vi "AK Befehl Auswerten_v1.3.vi"(10 "Array":string[](array[string])) -> (2 "String für schreiben":string)   [LabVIEW 2020, in "AK-Schnittstelle.lvlib"]
uses:
  AK-Schnittstelle.lvlib
  Aktionen Stoernummern pruefen.ctl
  Aktionen Zustandsfehlerinformation.ctl
  AK Namen Aktionen.ctl
  Seiten/FT-IR/Aktion FGV Rezepte wechseln.ctl
  Seiten/FT-IR/AK-manuell.ctl
  Seiten/System Einstellungen V2/Aktioen FGV System Konstanten.ctl
  Aktionen Gespeicherte Werte.ctl
  Seiten/System Einstellungen V2/Aktioen FGV System.ctl
  Funktionstasten/Funktionstasten-Aktion.ctl
  Funktionstasten/Zustaende.ctl
  Schedule Modul/Aktion FGV Scheduler Status.ctl
  Seiten/FT-IR/FGV FT-IR Aktionen.ctl
  Seiten/FT-IR/FGV FT-IR Diagnose Aktionen.ctl
  Seiten/Erweiterte Konfig/Status Dichtheitstest Aktionen.ctl
  Seiten/Erweiterte Konfig/FGV PID Aktionen.ctl
  Seiten/Anlagengrenzwerte/FGV Anlagengrenzwerte Aktionen.ctl
  Funktionstasten/Betriebsart.ctl
  Seiten/Log Konfig/Aktionen Trigger.ctl
  Messdaten/Aktionen FGV Messdaten.ctl
  Seiten/FT-IR/TOOLweb Interface Library/TOOLweb Rezept wechseln.vi
  Seiten/Erweiterte Konfig/Dichtheitstest.vi
  Funktionstasten/Funktionstasten.lvlib
  Seiten/Log Konfig/LogKonfig.lvlib
  Seiten/FT-IR/FT-IR.lvlib
  Seiten/FT-IR/FGV FT-IR Gasliste Aktionen.ctl
  Messdaten/Messdaten.lvlib
  Seiten/System Einstellungen V2/System Einstellungen V2.lvlib
  Seiten/Erweiterte Konfig/Erweiterte Konfig.lvlib
  Allgemein/allgemeine Sub-VIs.lvlib
  cRIO/PC/Kommunikation mit cRIO.lvlib
  Seiten/Anlagengrenzwerte/Anlagengrenzwerte.lvlib
  Seiten/FT-IR/TOOLweb Interface Library/TOOLweb Interface.lvlib
  Schedule Modul/Schedule Modul.lvlib
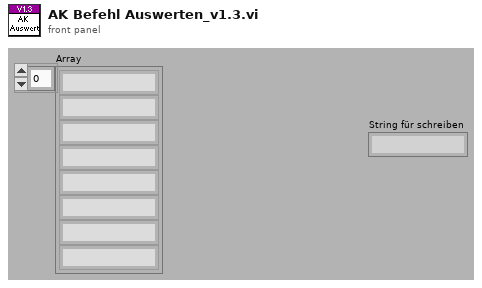
[diagram p1: front panel]
types:
  T1 = typedef "AK-Schnittstelle.lvlib/Aktionen Stoernummern pruefen.ctl" = enum16{"lesen", "prüfen"}
  T2 = typedef "AK-Schnittstelle.lvlib/Aktionen Zustandsfehlerinformation.ctl" = enum16{"OK", "Offline", "Busy", "Syntax Error", "Datenfehler"}
  T3 = typedef "AK-Schnittstelle.lvlib/AK Namen Aktionen.ctl" = enum16{"lesen", "laden", "speichern Namen", "AK Namen", "Liste erstellen", "EKFG erstellen", "speichern EKFG", "EKFG schreiben", "Neuen Eintrag erzeugen"}
  T4 = typedef "FT-IR.lvlib/AK-manuell.ctl" = enum16{"manuell", "Diesel", "CNG", "Gasoline"}
  T5 = typedef "FT-IR.lvlib/Aktion FGV Rezepte wechseln.ctl" = enum16{"lesen", "Rezepte", "Rezeptindex", "Diesel", "Gasoline", "NCG", "laden", "speichern", "AK/Man"}
  T6 = typedef "System Einstellungen V2.lvlib/Aktioen FGV System Konstanten.ctl" = enum16{"lesen", "laden", "speichern", "Sprache"}
  T7 = typedef "System Einstellungen V2.lvlib/Aktioen FGV System.ctl" = enum16{"lesen", "laden", "speichern", "Optionen schreiben", "Zeitstempel", "Reset BMP", "Reset SQP", "Wartung", "Werkseinstellung"}
  T8 = typedef "AK-Schnittstelle.lvlib/Aktionen Gespeicherte Werte.ctl" = enum16{"lesen", "laden", "speichern", "Seriell", "TCP", "Diverse", "AKTIV", "AK-Namen"}
  T9 = typedef "Messdaten.lvlib/Aktionen FGV Messdaten.ctl" = enum16{"lesen", "schreiben", "löschen", "Mittelwerte", "Komponente"}
  T10 = typedef "Funktionstasten.lvlib/Zustaende.ctl" = enum16{"Standby", "Pause", "Eco", "Messen", "Kalibrieren", "Spülen Filter", "Spülen Leitung", "Umgebungsluft", "0-Gas", "Cal-Gas", "CG zu PNS", "-------------", "Init 1", "Init 2", "Init 3", "Init 4", "Messen vorbereiten", "Messen durchführen", "Exit"}
  T11 = typedef "Funktionstasten.lvlib/Funktionstasten-Aktion.ctl" = enum16{"Initialisieren", "Zustand setzen", "Taste gedrückt", "Fehler speichern", "Lesen", "Manuell", "Remote", "Bitparallel", "Samplepoint", "Zeit Prüfen", "reset Umschalten"}
  T12 = typedef "Schedule Modul.lvlib/Aktion FGV Scheduler Status.ctl" = enum16{"lesen", "init", "aktiv", "inaktiv"}
  T13 = typedef "FT-IR.lvlib/FGV FT-IR Aktionen.ctl" = enum16{"lesen", "NOG setzen", "NOS setzen", "Initialisieren", "speichern", "ALLES setzen", "FT-IR Spektrum loggen", "Komm Stoppen", "Spektrum LogKonfig"}
  T14 = typedef "FT-IR.lvlib/FGV FT-IR Gasliste Aktionen.ctl" = enum16{"lesen", "Gasliste FT-IR", "Gasliste ausgelesen", "laden", "speichern", "löschen"}
  T15 = typedef "FT-IR.lvlib/FGV FT-IR Diagnose Aktionen.ctl" = enum16{"Lesen", "Diagnose Schreiben", "Min Schreiben", "Max Schreiben"}
  T16 = typedef "Erweiterte Konfig.lvlib/Status Dichtheitstest Aktionen.ctl" = enum16{"lesen", "Zeitstempel", "Daten", "läuft", "Protokolldaten"}
  T17 = typedef "Erweiterte Konfig.lvlib/FGV PID Aktionen.ctl" = enum16{"Lesen", "Schreiben PID", "Schreiben Sonstige", "Dichtheitstest", "Aktionen Dicht.", "Parameter Sensor"}
  T18 = typedef "Anlagengrenzwerte.lvlib/FGV Anlagengrenzwerte Aktionen.ctl" = enum16{"Lesen", "Grenzwerte schreiben"}
  T19 = typedef "Funktionstasten.lvlib/Betriebsart.ctl" = enum16{"Manuell", "Remote", "Bitparallel"}
  T20 = typedef "LogKonfig.lvlib/Aktionen Trigger.ctl" = enum16{"lesen", "ALLE schreiben", "Trigger prüfen", "Trigger rücksetzen"}
  T21 = cluster{"Modell":string, "ProjektNummer":string, "Software Version":string, "Seriennummer":string}
  T22 = typedef "System Einstellungen V2.lvlib/Optionen.ctl" = cluster{"Störmeldep.":bool, "Betriebszustände":bool, "AK in ppm":bool, "log Cal-Gas":bool, "log 0-Gas":bool, "Durchflusssensor 0-5V":bool, "PNS?":bool, "Mit N2 spülen":bool, "TRE08":bool, "Amium 10-Fach":bool, "Verticale Scrollbar aktiv":bool, "Loggingtakt":bool, "AK Rezeptwechsel gleich wie MKS":bool, "NG ECO":bool}
  T23 = typedef "AK-Schnittstelle.lvlib/Diverse gespeicherte Werte.ctl" = cluster{"Kalibriergaseingang":i16, "SamplePoint":i16, "CalGas zu PNS":i16, "Gas-Reihenfolge":i16[], "Zeit 0-Gas":sgl, "Zeit CalGas":sgl, "AK Befehlssatz":T24}
  T24 = typedef "AK-Schnittstelle.lvlib/AK Befehlssatz.ctl" = enum16{"MEXA", "IAG v1.4", "AVL (Puma)", "PEUS"}
  T25 = typedef "String - Ausgabefeld.ctl" = string
  T26 = typedef "Verwaltung - cRIO.lvlib/TC Eingaenge.ctl" = cluster{"TC0: Reserve":sgl, "TC1: HL zu FT-IR":sgl, "TC2: HL Extern SP1":sgl, "TC3: HL Extern SP2":sgl, "TC4: Reserve":sgl, "TC5: Reserve":sgl, "TC6: Reserve":sgl, "TC7: Reserve":sgl, "TC8: FT-IR":sgl, "TC9: Reserve":sgl, "TC10: Schaltschrank":sgl, "TC11: Umgebung":sgl}
  T27 = typedef "Verwaltung - cRIO.lvlib/Analog Eingaenge.ctl" = cluster{"AI0: Durchfluss FT-IR":sgl, "AI1: Druck Ausgang":sgl, "AI2: Umgebungsdruck":sgl, "AI3: Druck FT-IR":sgl, "AI4: Druck CalGas":sgl, "AI5: Reserve":sgl, "AI6: Reserve":sgl, "AI7: Reserve":sgl, "Rohwert Durchfluss FT-IR":sgl, "Rohwert Druck Ausgang":sgl, "Rohwert Umgebungsdruck":sgl, "Rohwert Druck FT-IR":sgl, "Rohwert Druck CalGas":sgl, "Rohwert AI5":sgl, "Rohwert AI6":sgl, "Rohwert AI7":sgl, "Rohwert Diffdruck mbar FTIR":sgl}
  T28 = typedef "Erweiterte Konfig.lvlib/Sonstige Parameter.ctl" = cluster{"Lüfter langsam":sgl, "Lüfter schnell":sgl, "FT-IR Kühlung Soll":sgl, "FT-IR Kühlung Max":sgl, "Überwachung":T29, "Befüllung aktiv":T30, "Stickstoff Befüllzeit":sgl, "Befüllintervall":sgl, "Kalibrierwert FT-IR":sgl, "Offset Ausgang":sgl, "Offset FT-IR":sgl, "Offset Druck FT-IR":sgl, "Dichtheitstest Zeit":sgl, "Dichtheitstest Abfall":sgl, "Dichtheitstest Umfang":T31, "Offset Umgebung":sgl, "Max Taupunkt":sgl, "Pumpendrehzahl":sgl, "ext. Befüllung":T30, "Ext. Stickstoff Befüllzeit":sgl}
  T29 = typedef "Auswahlfeld.ctl" = u16
  T30 = typedef "LogKonfig.lvlib/Auswahlfeld aktiviert-deaktiviert.ctl" = u16
  T31 = typedef "Erweiterte Konfig.lvlib/Dichtheitstest Umfang.ctl" = u16
  T32 = typedef "Anlagengrenzwerte.lvlib/Anlagen-Grenzwerte Anzeige.ctl" = cluster{"Eingangsdruck FT-IR:":T33, "Durchfluss FT-IR:":T33, "Durchfluss CalGas:":T33, "Druck Ausgang:":T33, "Druck Kalter Block:":T33, "Heizleitungen intern:":T33, "Heizleitung zu FT-IR:":T33, "Heizung Filterblock:":T33, "Heizung Pumpe:":T33, "Heizleitung Extern SP1:":T33, "Heizleitung Extern SP2:":T33, "FT-IR Heizung Messzelle:":T33, "Schaltschranktemperatur:":T33, "Gaskühler:":T33}
  T33 = typedef "Anlagengrenzwerte.lvlib/Anlagen-Parameter Anzeige.ctl" = cluster{"Sollwert":sgl, "Warn-Min":sgl, "Warn-Max":sgl, "Abschalt-Min":sgl, "Abschalt-Max":sgl, "Regler":u16}
  T34 = typedef "LogKonfig.lvlib/Element Triggerereignisse.ctl" = cluster{"Trigger verwenden":T30, "Messwert":u16, "kl./gr.":u16, "Wert":sgl, "Puffergröße":sgl}
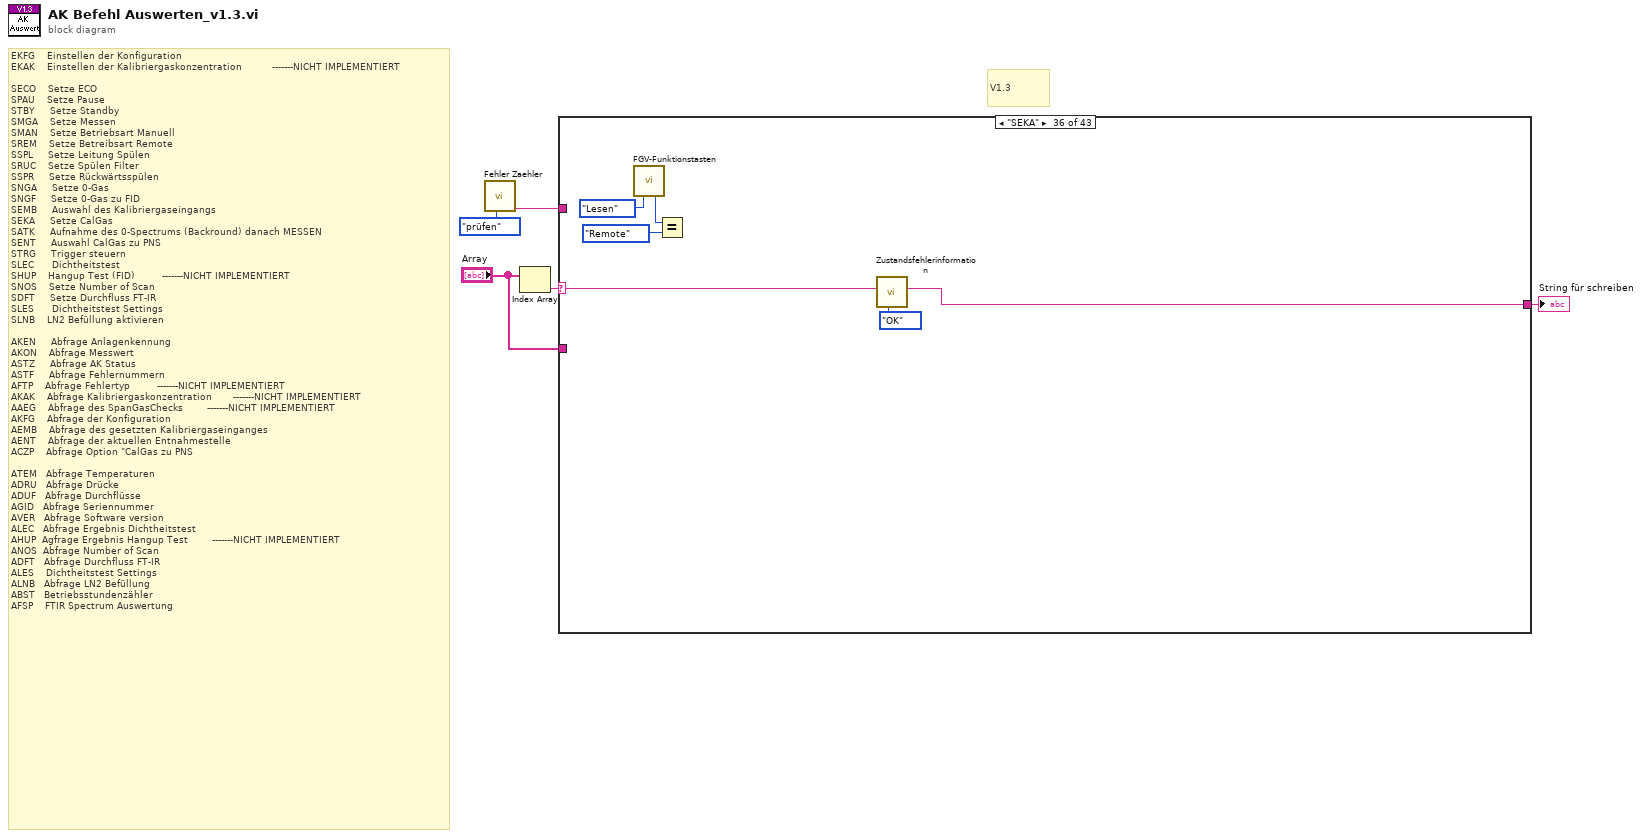
[diagram p0: block diagram]
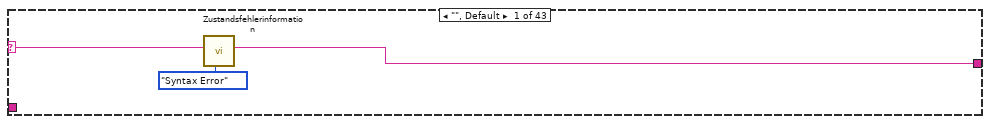
[diagram p2: hidden frame]
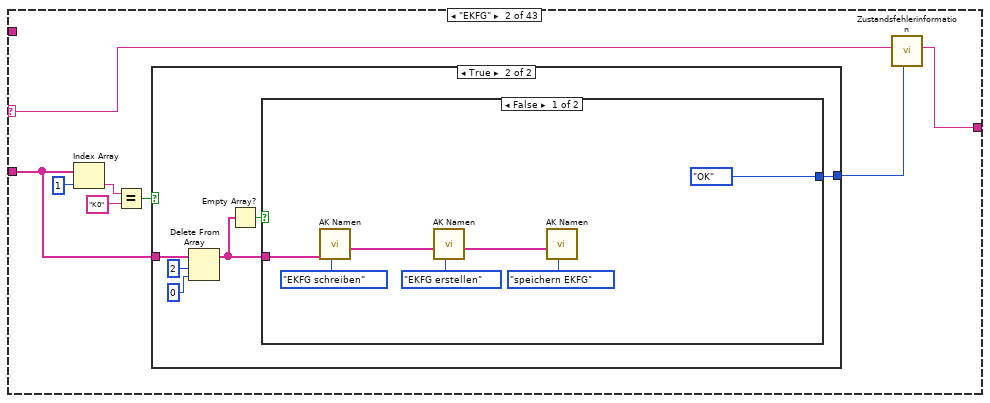
[diagram p3: hidden frame]
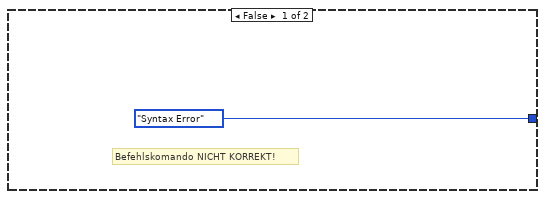
[diagram p4: hidden frame]
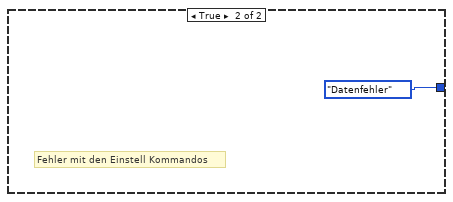
[diagram p5: hidden frame]
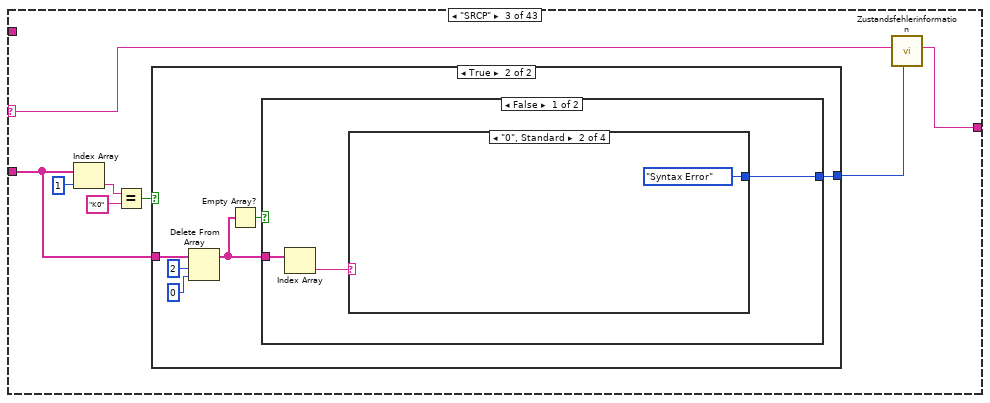
[diagram p6: hidden frame]
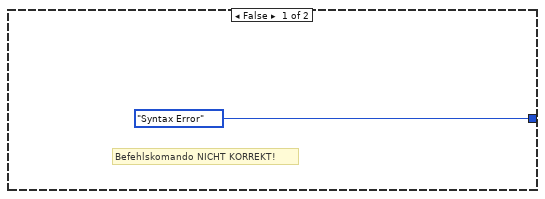
[diagram p7: hidden frame]
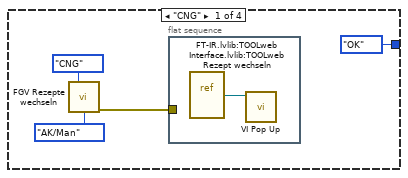
[diagram p8: hidden frame]
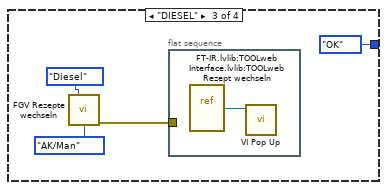
[diagram p9: hidden frame]
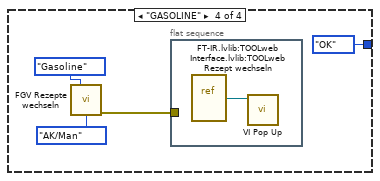
[diagram p10: hidden frame]
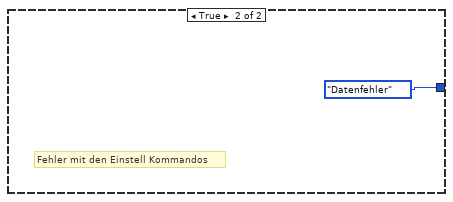
[diagram p11: hidden frame]
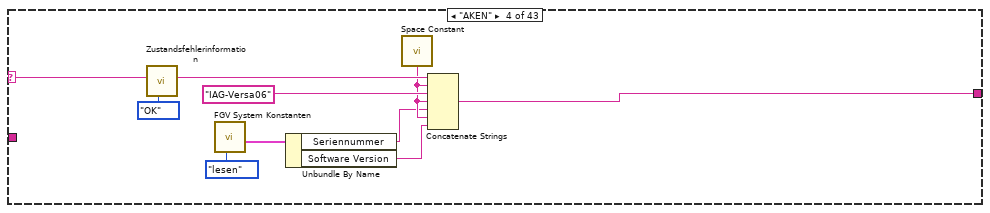
[diagram p12: hidden frame]
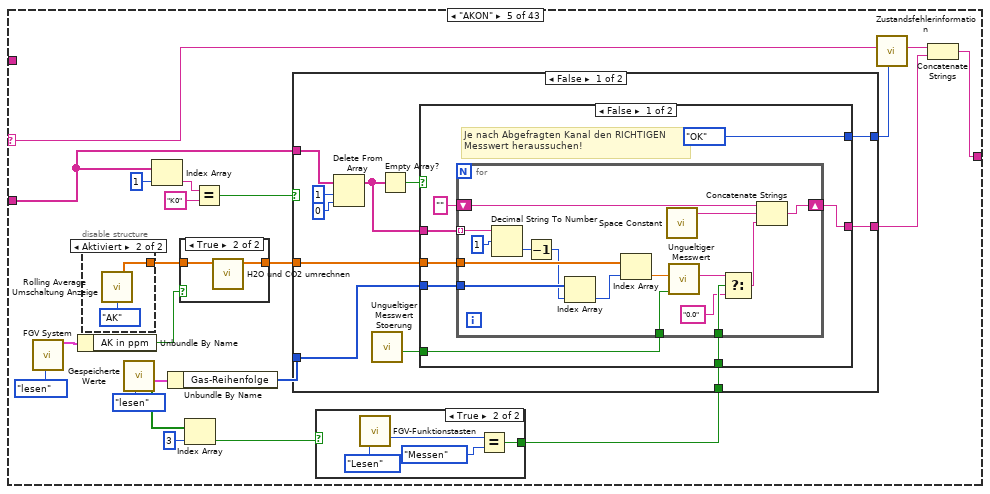
[diagram p13: hidden frame]
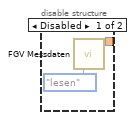
[diagram p14: hidden frame]
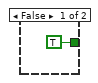
[diagram p15: hidden frame]
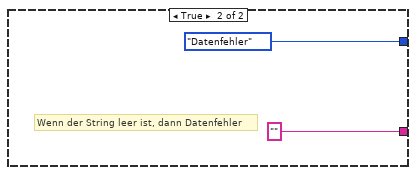
[diagram p17: hidden frame]
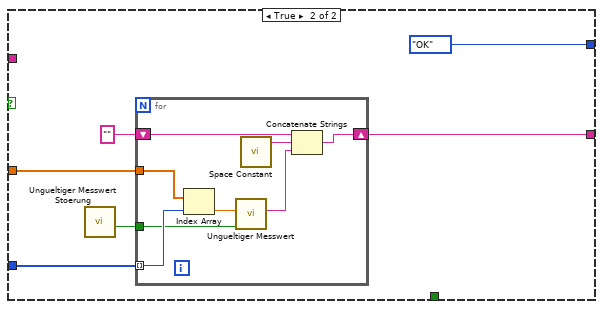
[diagram p18: hidden frame]
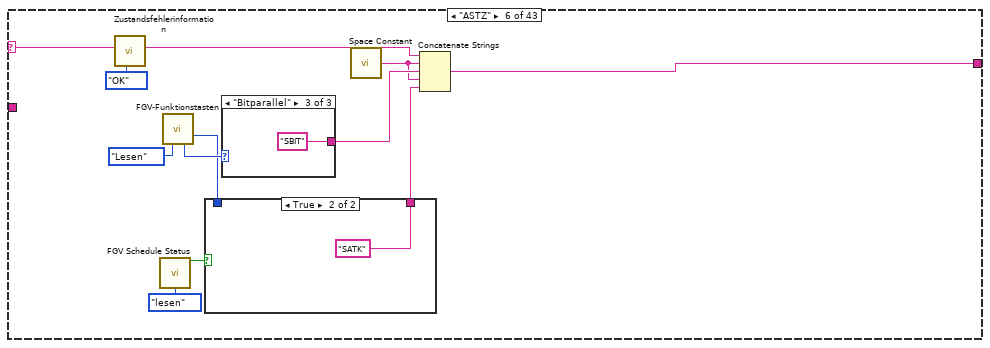
[diagram p19: hidden frame]
diagram:
  # "V1.3"
  # "EKFG    Einstellen der Konfiguration\nEKAK    Einstellen der Kalibriergaskonzentration          -------NICHT IMPLEMENTIERT\n\nSECO    Setze ECO\nSPAU    Setze Pause\nSTBY     Setze Standby\nSMGA    Setze Messen\nSMAN    Setze Betriebsart Manuell\nSREM    Setze Betreibsart Remote\nSSPL     Setze Leitung Spülen\nSRUC    Setze Spülen Filter\nSSPR     Setze Rückwärtsspülen\nSNGA     Setze 0-Gas\nSNGF     Setze 0-Gas zu FID\nSEMB     Auswahl des Kalibriergaseingangs\nSEKA     Setze CalGas\nSATK     Aufnahme des 0-Spectrums (Backround) danach MESSEN\nSENT     Auswahl CalGas zu PNS\nSTRG     Trigger steuern\nSLEC      Dichtheitstest\nSHUP    Hangup Test (FID)         -------NICHT IMPLEMENTIERT\nSNOS    Setze Number of Scan\nSDFT     Setze Durchfluss FT-IR\nSLES      Dichtheitstest Settings\nSLNB    LN2 Befüllung aktivieren\n\nAKEN     Abfrage Anlagenkennung\nAKON    Abfrage Messwert\nASTZ     Abfrage AK Status\nASTF     Abfrage Fehlernummern\nAFTP    Abfrage Fehlertyp         -------NICHT IMPLEMENTIERT\nAKAK    Abfrage Kalibriergaskonzentration       -------NICHT IMPLEMENTIERT\nAAEG    Abfrage des SpanGasChecks        -------NICHT IMPLEMENTIERT\nAKFG    Abfrage der Konfiguration\nAEMB    Abfrage des gesetzten Kalibriergaseinganges\nAENT    Abfrage der aktuellen Entnahmestelle\nACZP    Abfrage Option \"CalGas zu PNS\n\nATEM   Abfrage Temperaturen\nADRU   Abfrage Drücke\nADUF   Abfrage Durchflüsse\nAGID   Abfrage Seriennummer\nAVER   Abfrage Software version\nALEC   Abfrage Ergebnis Dichtheitstest\nAHUP  Agfrage Ergebnis Hangup Test        -------NICHT IMPLEMENTIERT\nANOS  Abfrage Number of Scan\nADFT   Abfrage Durchfluss FT-IR\nALES    Dichtheitstest Settings\nALNB   Abfrage LN2 Befüllung\nABST   Betriebsstundenzähler\nAFSP    FTIR Spectrum Auswertung"
  n1 = call "Fehler Zaehler.vi"("Aktionen"=Aktionen_Stoernummern_pruefen."prüfen") -> ("Fehlerzähler"=w3:string)  [unwired: 7 in, 3 out]
  n2 = Index Array(array="Array") -> (element=w2:string)  [unwired: 1 in]
  n3 = case shown="\"SEKA\"" w2 {
    selector: w2 -> [w7 w15 w38 w74 w97 w171 w194 w201 w212 w242 w250 w259 w277 w300 w314 w321 w329 w344 w365 w376 w385 w395 w409 w417 w420 w423 w426 w436 w446 w450 w460 w464 w466 w479 w484 w506 w511 w515 w537 w576 w600 w651 w682]
    tunnel: [w6 w14 w37 w76 w98 w173 w196 w203 w214 w244 w252 w261 w267 w295 w311 w316 w325 w337 w363 w378 w387 w397 w407 w416 w419 w422 w425 w435 w445 w449 w459 w463 w465 w478 w483 w505 w510 w514 w536 w575 w599 w650 w681] -> w5
    tunnel: w3 -> [_ _ _ _ _ _ _ _ _ _ _ _ _ _ _ _ _ _ _ _ _ _ _ _ _ _ _ _ _ _ _ _ _ _ _ _ _ _ _ _ _ _ _]
    tunnel: "Array" -> [_ w16 w39 _ w88 _ _ _ _ _ _ _ _ _ _ _ _ _ _ _ _ _ _ _ _ _ _ w428 w438 _ w458 _ _ _ w482 _ _ w513 w535 _ w598 w649 w680]
    frame "", Default {
      n4 = call "Zustandsfehlerinformation.vi"("Aktionen"=Aktionen_Zustandsfehlerinformation."Syntax Error", "String"=w7) -> ("String"=w6:string)  [unwired: 9 in]
    }
    frame "EKFG" {
      n5 = Index Array(array=w16, index=1 ("Index")) -> (element=w12:string)
      n6 = Equal?(x=w12, y="K0") -> (x = y?=w10:bool)
      n7 = case shown="True" w10 {
        tunnel: w16 -> [_ w21]
        tunnel: [Aktionen_Zustandsfehlerinformation."Syntax Error" ("Aktionen") w18] -> w9
        frame False {
          # "Befehlskomando NICHT KORREKT!"
        }
        frame True {
          n8 = Delete From Array(array=w21, length=2 ("Länge"), index=0 ("Index")) -> (array with subset deleted=w20:string[])  [unwired: 1 out]
          n9 = Empty Array?(array=w20) -> (empty?=w19:bool)
          n10 = case shown="False" w19 {
            tunnel: w20 -> [w29 _]
            tunnel: [Aktionen_Zustandsfehlerinformation."OK" ("Aktionen") Aktionen_Zustandsfehlerinformation."Datenfehler" ("Aktionen")] -> w18
            frame False {
              n11 = call "AK Namen.vi"("Aktionen"=AK_Namen_Aktionen."EKFG schreiben", "EKFG Liste"=w29) -> ("AK Namen"=w26:string[])  [unwired: 6 in, 3 out]
              n12 = call "AK Namen.vi"("Aktionen"=AK_Namen_Aktionen."EKFG erstellen", "AK Namen"=w26) -> ("AK Namen"=w24:string[])  [unwired: 6 in, 3 out]
              n13 = call "AK Namen.vi"("Aktionen"=AK_Namen_Aktionen."speichern EKFG", "AK Namen"=w24) -> ()  [unwired: 6 in, 4 out]
            }
            frame True {
              # "Fehler mit den Einstell Kommandos"
            }
          }
        }
      }
      n14 = call "Zustandsfehlerinformation.vi"("Aktionen"=w9, "String"=w15) -> ("String"=w14:string)  [unwired: 9 in]
    }
    frame "SRCP" {
      n15 = Index Array(array=w39, index=1 ("Index")) -> (element=w35:string)
      n16 = Equal?(x=w35, y="K0") -> (x = y?=w33:bool)
      n17 = case shown="True" w33 {
        tunnel: w39 -> [_ w44]
        tunnel: [Aktionen_Zustandsfehlerinformation."Syntax Error" ("Aktionen") w41] -> w32
        frame False {
          # "Befehlskomando NICHT KORREKT!"
        }
        frame True {
          n18 = Delete From Array(array=w44, length=2 ("Länge"), index=0 ("Index")) -> (array with subset deleted=w43:string[])  [unwired: 1 out]
          n19 = Empty Array?(array=w43) -> (empty?=w42:bool)
          n20 = case shown="False" w42 {
            tunnel: w43 -> [w48 _]
            tunnel: [w49 Aktionen_Zustandsfehlerinformation."Datenfehler" ("Aktionen")] -> w41
            frame False {
              n21 = Index Array(array=w48) -> (element=w47:string)  [unwired: 1 in]
              n22 = case shown="\"0\", Standard" w47 {
                tunnel: [Aktionen_Zustandsfehlerinformation."OK" ("Aktionen") Aktionen_Zustandsfehlerinformation."Syntax Error" ("Aktionen") Aktionen_Zustandsfehlerinformation."OK" ("Aktionen") Aktionen_Zustandsfehlerinformation."OK" ("Aktionen")] -> w49
                frame "CNG" {
                  n23 = call "FGV Rezepte wechseln.vi"("AK/man"=AK-manuell."CNG", "Aktion"=Aktion_FGV_Rezepte_wechseln."AK/Man") -> ("error out"=w52:errorcluster)  [unwired: 7 in, 6 out]
                  n24 = flat-sequence {
                    tunnel: w52 -> [_]
                    frame #0 {
                      n25 = vi-ref "FT-IR.lvlib:TOOLweb Interface.lvlib:TOOLweb Rezept wechseln.vi"() -> (w54:refnum<vi>)
                      n26 = call "VI Pop Up.vi"("VI Referenz"=w54) -> ()  [unwired: 10 in, 1 out]
                    }
                  }
                }
                frame "0", Default {
                }
                frame "DIESEL" {
                  n27 = call "FGV Rezepte wechseln.vi"("AK/man"=AK-manuell."Diesel", "Aktion"=Aktion_FGV_Rezepte_wechseln."AK/Man") -> ("error out"=w58:errorcluster)  [unwired: 7 in, 6 out]
                  n28 = flat-sequence {
                    tunnel: w58 -> [_]
                    frame #0 {
                      n29 = vi-ref "FT-IR.lvlib:TOOLweb Interface.lvlib:TOOLweb Rezept wechseln.vi"() -> (w60:refnum<vi>)
                      n30 = call "VI Pop Up.vi"("VI Referenz"=w60) -> ()  [unwired: 10 in, 1 out]
                    }
                  }
                }
                frame "GASOLINE" {
                  n31 = call "FGV Rezepte wechseln.vi"("AK/man"=AK-manuell."Gasoline", "Aktion"=Aktion_FGV_Rezepte_wechseln."AK/Man") -> ("error out"=w63:errorcluster)  [unwired: 7 in, 6 out]
                  n32 = flat-sequence {
                    tunnel: w63 -> [_]
                    frame #0 {
                      n33 = vi-ref "FT-IR.lvlib:TOOLweb Interface.lvlib:TOOLweb Rezept wechseln.vi"() -> (w65:refnum<vi>)
                      n34 = call "VI Pop Up.vi"("VI Referenz"=w65) -> ()  [unwired: 10 in, 1 out]
                    }
                  }
                }
              }
            }
            frame True {
              # "Fehler mit den Einstell Kommandos"
            }
          }
        }
      }
      n35 = call "Zustandsfehlerinformation.vi"("Aktionen"=w32, "String"=w38) -> ("String"=w37:string)  [unwired: 9 in]
    }
    frame "AKEN" {
      n36 = call "Zustandsfehlerinformation.vi"("Aktionen"=Aktionen_Zustandsfehlerinformation."OK", "String"=w74) -> ("String"=w73:string)  [unwired: 9 in]
      n37 = call "FGV System Konstanten.vi"("Aktionen"=Aktioen_FGV_System_Konstanten."lesen") -> ("Cluster out"=w69:T21)  [unwired: 6 in, 4 out]
      n38 = Unbundle By Name(w69) -> ("Seriennummer"=w68:string, "Software Version"=w67:string)
      n39 = call <vilib>:"Space Constant.vi"() -> ("String"=w70:string)
      n40 = Concatenate Strings(w73, w70, "IAG-Versa06" ("String"), w70, w68, w70, w67) -> (w76:string)
    }
    frame "AKON" {
      n41 = call "FGV System.vi"("Aktionen"=Aktioen_FGV_System."lesen") -> ("Optionen"=w83:T22)  [unwired: 12 in, 6 out]
      n42 = Unbundle By Name(w83) -> ("AK in ppm"=w85:bool)
      n43 = disable-structure shown="Aktiviert" {
        disable-tunnel: [w100 w102] -> w77
        frame Disabled {
          n44 = call "FGV Messdaten.vi"("Aktionen"=Aktionen_FGV_Messdaten."lesen") -> ("Aktuelle Messwerte"=w100:sgl[])  [unwired: 6 in, 8 out]
        }
        frame Enabled {
          n45 = call "Rolling Average Umschaltung Anzeige.vi"("Aktion"=enum16{"AK", "IAG Software"}."AK") -> ("Aktuelle Messwerte"=w102:sgl[])  [unwired: 9 in, 5 out]
        }
      }
      n46 = call "Gespeicherte Werte.vi"("Aktionen"=Aktionen_Gespeicherte_Werte."lesen") -> ("AKTIV?"=w80:bool[], "Diverse Werte"=w86:T23)  [unwired: 6 in, 3 out]
      n47 = Index Array(array=w88, index=1 ("Index")) -> (element=w91:string)
      n48 = Unbundle By Name(w86) -> ("Gas-Reihenfolge"=w94:i16[])
      n49 = case shown="True" w85 {
        tunnel: w77 -> [w108 w110]
        tunnel: [w108 w109] -> w82
        frame False {
        }
        frame True {
          n50 = call "H2O und CO2 umrechnen.vi"("Aktuelle Messwerte"=w110) -> ("Aktuelle Messwerte"=w109:sgl[])  [unwired: 10 in]
        }
      }
      n51 = Index Array(array=w80, index=3 ("Index")) -> (element=w78:bool)
      n52 = Equal?(x=w91, y="K0") -> (x = y?=w89:bool)
      n53 = case shown="True" w78 {
        tunnel: [TRUE w104] -> w81
        frame False {
        }
        frame True {
          n54 = call "FGV-Funktionstasten.vi"("Aktion"=Funktionstasten-Aktion."Lesen") -> ("ausgewählte Funktion"=w106:T10)  [unwired: 7 in, 7 out]
          n55 = Equal?(x=w106, y=Zustaende."Messen") -> (x = y?=w104:bool)
        }
      }
      n56 = case shown="False" w89 {
        tunnel: w94 -> [w115 w153]
        tunnel: [w113 w151] -> w93
        tunnel: w82 -> [w114 w150]
        tunnel: w88 -> [w119 _]
        tunnel: [w117 Aktionen_Zustandsfehlerinformation."OK" ("Aktionen")] -> w87
        tunnel: w81 -> [w111 _]
        frame False {
          n57 = Delete From Array(array=w119, length=1 ("Länge"), index=0 ("Index")) -> (array with subset deleted=w116:string[])  [unwired: 1 out]
          n58 = call "Ungueltiger Messwert Stoerung.vi"() -> ("Störung Messgerät"=w112:bool)  [unwired: 11 in]
          n59 = Empty Array?(array=w116) -> (empty?=w118:bool)
          n60 = case shown="False" w118 {
            tunnel: [Aktionen_Zustandsfehlerinformation."OK" ("Aktionen") Aktionen_Zustandsfehlerinformation."Datenfehler" ("Aktionen")] -> w117
            tunnel: w116 -> [w128 _]
            tunnel: w115 -> [w127 _]
            tunnel: w114 -> [w126 _]
            tunnel: [w125 ""] -> w113
            tunnel: w112 -> [w123 _]
            tunnel: w111 -> [w122 _]
            frame False {
              # "Je nach Abgefragten Kanal den RICHTIGEN\nMesswert heraussuchen!"
              n61 = for {
                tunnel: w128 -> [w145] mode=indexing
                tunnel: w127 -> [w143]
                tunnel: w126 -> [w142]
                shift-right: [w141] -> w125
                shift-left: "" -> [w140]
                tunnel: w123 -> [w134]
                tunnel: w122 -> [w132]
                n62 = Decimal String To Number(string=w145, offset=1 ("Offset (0)")) -> (number=w139:i32)  [unwired: 1 in, 1 out]
                n63 = Decrement(x=w139) -> (x-1=w138:i32)
                n64 = Index Array(array=w143, index=w138) -> (element=w136:i16)
                n65 = Index Array(array=w142, index=w136) -> (element=w135:sgl)
                n66 = call <vilib>:"Space Constant.vi"() -> ("String"=w137:string)
                n67 = call "Ungueltiger Messwert.vi"("Stöung Messgerät"=w134, "Messwert"=w135) -> ("Messwert String"=w131:string)  [unwired: 9 in]
                n68 = Select(t=w131, s=w132, f="0.0") -> (s? t:f=w133:string)
                n69 = Concatenate Strings(w140, w137, w133) -> (w141:string)
              }
            }
            frame True {
              # "Wenn der String leer ist, dann Datenfehler"
            }
          }
        }
        frame True {
          n70 = call "Ungueltiger Messwert Stoerung.vi"() -> ("Störung Messgerät"=w148:bool)  [unwired: 11 in]
          n71 = for {
            tunnel: w153 -> [w157] mode=indexing
            shift-right: [w161] -> w151
            shift-left: "" -> [w160]
            tunnel: w150 -> [w159]
            tunnel: w148 -> [w155]
            n72 = Index Array(array=w159, index=w157) -> (element=w156:sgl)
            n73 = call "Ungueltiger Messwert.vi"("Stöung Messgerät"=w155, "Messwert"=w156) -> ("Messwert String"=w154:string)  [unwired: 9 in]
            n74 = call <vilib>:"Space Constant.vi"() -> ("String"=w158:string)
            n75 = Concatenate Strings(w160, w158, w154) -> (w161:string)
          }
        }
      }
      n76 = call "Zustandsfehlerinformation.vi"("Aktionen"=w87, "String"=w97) -> ("String"=w96:string)  [unwired: 9 in]
      n77 = Concatenate Strings(w96, w93) -> (w98:string)
    }
    frame "ASTZ" {
      n78 = call "Zustandsfehlerinformation.vi"("Aktionen"=Aktionen_Zustandsfehlerinformation."OK", "String"=w171) -> ("String"=w170:string)  [unwired: 9 in]
      n79 = call "FGV Schedule Status.vi"("Aktion"=Aktion_FGV_Scheduler_Status."lesen") -> ("Scheduler Status"=w164:bool)  [unwired: 13 in, 1 out]
      n80 = call "FGV-Funktionstasten.vi"("Aktion"=Funktionstasten-Aktion."Lesen") -> ("ausgewählte Funktion"=w162:T10, "Betriebsart"=w168:T19)  [unwired: 7 in, 6 out]
      n81 = case shown="True" w164 {
        tunnel: w162 -> [w175 _]
        tunnel: [w174 "SATK" ("String")] -> w163
        frame False {
          n82 = case shown="\"Init 4\"" w175 {
            tunnel: ["STBY" ("String") "SPAU" ("String") "SECO" ("String") "SMGA" ("String") "SATK" ("String") "SEKA" ("String") "SRUC" ("String") "SSPL" ("String") "SNGA" ("String") "SCZP" ("String") _ _ _ _ _ _ _ _] -> w174
            frame "Standby", Default {
            }
            frame "Pause" {
            }
            frame "Eco" {
            }
            frame "Messen" {
            }
            frame "Kalibrieren" {
            }
            frame "Cal-Gas" {
              # "#KaliAutoMessenBug"
            }
            frame "Spülen Filter" {
            }
            frame "Spülen Leitung" {
            }
            frame "0-Gas" {
            }
            frame "CG zu PNS" {
              # "#KaliAutoMessenBug"
            }
            frame "Init 1" {
            }
            frame "Init 2" {
            }
            frame "-------------" {
            }
            frame "Init 3" {
            }
            frame "Init 4" {
            }
            frame "Messen vorbereiten" {
            }
            frame "Messen durchführen" {
            }
            frame "Exit" {
            }
          }
        }
        frame True {
        }
      }
      n83 = case shown="\"Bitparallel\"" w168 {
        tunnel: ["SMAN" ("String") "SREM" ("String") "SBIT" ("String")] -> w167
        frame "Manuell", Default {
        }
        frame "Remote" {
        }
        frame "Bitparallel" {
        }
      }
      n84 = call <vilib>:"Space Constant.vi"() -> ("String"=w166:string)
      n85 = Concatenate Strings(w170, w166, w167, w166, w163) -> (w173:string)
    }
    frame "ARCP" {
      n86 = call "Zustandsfehlerinformation.vi"("Aktionen"=Aktionen_Zustandsfehlerinformation."OK", "String"=w194) -> ("String"=w193:string)  [unwired: 9 in]
      n87 = call "FGV FT-IR Parameter.vi"("Aktion"=FGV_FT-IR_Aktionen."lesen") -> ("Current Recipe"=w190:string)  [unwired: 11 in, 7 out]
      n88 = call <vilib>:"Space Constant.vi"() -> ("String"=w192:string)
      n89 = Concatenate Strings(w193, w192, w190) -> (w196:string)
    }
    frame "ASTF" {
      n90 = call "Zustandsfehlerinformation.vi"("Aktionen"=Aktionen_Zustandsfehlerinformation."OK", "String"=w201) -> ("String"=w200:string)  [unwired: 9 in]
      n91 = call "Fehler Zaehler.vi"("Aktionen"=Aktionen_Stoernummern_pruefen."lesen") -> ("Fehler Nummern"=w198:string)  [unwired: 7 in, 3 out]
      n92 = call <vilib>:"Space Constant.vi"() -> ("String"=w197:string)
      n93 = Concatenate Strings(w200, w197, w198) -> (w203:string)
    }
    frame "AKFG" {
      n94 = call "Gespeicherte Werte.vi"("Aktionen"=Aktionen_Gespeicherte_Werte."lesen") -> ("Diverse Werte"=w208:T23)  [unwired: 6 in, 4 out]
      n95 = Unbundle By Name(w208) -> ("Gas-Reihenfolge"=w210:i16[])
      n96 = disable-structure shown="Deaktiviert" {
        disable-tunnel: [w233 _] -> _
        frame Disabled {
          n97 = call "FGV Gasliste.vi"("Aktionen"=FGV_FT-IR_Gasliste_Aktionen."lesen") -> ("Aktuelle Gasliste gesamt"=w233:T25[])  [unwired: 8 in, 2 out]
        }
        frame Enabled {
        }
      }
      n98 = call "AK Namen.vi"("Aktionen"=AK_Namen_Aktionen."lesen") -> ("AK Namen"=w204:string[])  [unwired: 7 in, 3 out]
      n99 = for {
        tunnel: w210 -> [w223] mode=indexing
        shift-right: [w226] -> w207
        shift-left: "" -> [w225]
        tunnel: w204 -> [w224]
        i -> [w217]
        n100 = Index Array(array=w224, index=w223) -> (element=w221:string)
        n101 = for {
          N: 15 -> [_]
          shift-right: [w231] -> w220
          shift-left: w221 -> [w232]
          stop <- w229 stop-if-true
          n102 = call <vilib>:"Space Constant.vi"() -> ("String"=w228:string)
          n103 = Search and Replace String(input string=w232, search string=w228, replace string="_") -> (result string=w231:string, number of replacements=w230:i32)  [unwired: 5 in, 2 out]
          n104 = Less Or Equal To 0?(x=w230) -> (x <= 0?=w229:bool)
        }
        n105 = Increment(x=w217) -> (x+1=w216:i32)
        n106 = Number To Decimal String(number=w216) -> (decimal integer string=w215:string)  [unwired: 1 in]
        n107 = call <vilib>:"Space Constant.vi"() -> ("String"=w219:string)
        n108 = Concatenate Strings(w225, w219, w220, w219, "K" ("String"), w215) -> (w226:string)
      }
      n109 = call "Zustandsfehlerinformation.vi"("Aktionen"=Aktionen_Zustandsfehlerinformation."OK", "String"=w212) -> ("String"=w211:string)  [unwired: 9 in]
      n110 = Concatenate Strings(w211, w207) -> (w214:string)
    }
    frame "AEMB" {
      n111 = call "Zustandsfehlerinformation.vi"("Aktionen"=Aktionen_Zustandsfehlerinformation."OK", "String"=w242) -> ("String"=w241:string)  [unwired: 9 in]
      n112 = call "Gespeicherte Werte.vi"("Aktionen"=Aktionen_Gespeicherte_Werte."lesen") -> ("Diverse Werte"=w235:T23)  [unwired: 6 in, 4 out]
      n113 = Unbundle By Name(w235) -> ("Kalibriergaseingang"=w239:i16)
      n114 = call <vilib>:"Space Constant.vi"() -> ("String"=w236:string)
      n115 = Number To Decimal String(number=w239) -> (decimal integer string=w237:string)  [unwired: 1 in]
      n116 = Concatenate Strings(w241, w236, "M" ("String"), w237) -> (w244:string)
    }
    frame "AENT" {
      n117 = call "Zustandsfehlerinformation.vi"("Aktionen"=Aktionen_Zustandsfehlerinformation."OK", "String"=w250) -> ("String"=w249:string)  [unwired: 9 in]
      n118 = call "FGV-Funktionstasten.vi"("Aktion"=Funktionstasten-Aktion."Lesen") -> ("Samplepoint"=w245:u16)  [unwired: 7 in, 7 out]
      n119 = call <vilib>:"Space Constant.vi"() -> ("String"=w247:string)
      n120 = Number To Decimal String(number=w245) -> (decimal integer string=w248:string)  [unwired: 1 in]
      n121 = Concatenate Strings(w249, w247, w248) -> (w252:string)
    }
    frame "ACZP" {
      n122 = call "Zustandsfehlerinformation.vi"("Aktionen"=Aktionen_Zustandsfehlerinformation."OK", "String"=w259) -> ("String"=w258:string)  [unwired: 9 in]
      n123 = call "Gespeicherte Werte.vi"("Aktionen"=Aktionen_Gespeicherte_Werte."lesen") -> ("Diverse Werte"=w253:T23)  [unwired: 6 in, 4 out]
      n124 = Unbundle By Name(w253) -> ("CalGas zu PNS"=w256:i16)
      n125 = call <vilib>:"Space Constant.vi"() -> ("String"=w254:string)
      n126 = Number To Decimal String(number=w256) -> (decimal integer string=w255:string)  [unwired: 1 in]
      n127 = Concatenate Strings(w258, w254, w255) -> (w261:string)
    }
    frame "ATEM" {
      n128 = call "Zustandsfehlerinformation.vi"("Aktionen"=Aktionen_Zustandsfehlerinformation."OK", "String"=w277) -> ("String"=w266:string)  [unwired: 9 in]
      n129 = call "FGV cRIO-Daten.vi"("Aktion"=enum16{"lesen", "schreiben"}."lesen") -> ("TC Eingänge"=w262:T26)  [unwired: 9 in, 9 out]
      n130 = Unbundle By Name(w262) -> ("TC0: Reserve"=w273:sgl, "TC1: HL zu FT-IR"=w272:sgl, "TC2: HL Extern SP1"=w271:sgl, "TC3: HL Extern SP2"=w270:sgl, "TC4: Reserve"=w269:sgl, "TC5: Reserve"=w265:sgl, "TC6: Reserve"=w264:sgl, "TC7: Reserve"=w263:sgl)
      n131 = call "FGV FT-IR Diagnosewerte.vi"("Aktionen"=FGV_FT-IR_Diagnose_Aktionen."Lesen") -> ("Temperatur"=w274:dbl)  [unwired: 5 in, 5 out]
      n132 = Build Array(w274, w273, w272, w271, w270, w269, w265, w264, w263) -> (w268:dbl[])
      n133 = for {
        tunnel: w268 -> [w284] mode=indexing
        shift-right: [w279] -> w267
        shift-left: w266 -> [w282]
        n134 = Number To Fractional String(number=w284, precision (6)=i16 1 ("Genauigkeit (6)")) -> (F-format string=w280:string)  [unwired: 2 in]
        n135 = call <vilib>:"Space Constant.vi"() -> ("String"=w281:string)
        n136 = Concatenate Strings(w282, w281, w280) -> (w279:string)
      }
    }
    frame "ADRU" {
      n137 = call "Zustandsfehlerinformation.vi"("Aktionen"=Aktionen_Zustandsfehlerinformation."OK", "String"=w300) -> ("String"=w294:string)  [unwired: 9 in]
      n138 = call "FGV cRIO-Daten.vi"("Aktion"=enum16{"lesen", "schreiben"}."lesen") -> ("Analog Input"=w298:T27)  [unwired: 9 in, 9 out]
      n139 = Unbundle By Name(w298) -> ("AI1: Druck Ausgang"=w290:sgl, "AI3: Druck FT-IR"=w288:sgl)
      n140 = call "FGV FT-IR Diagnosewerte.vi"("Aktionen"=FGV_FT-IR_Diagnose_Aktionen."Lesen") -> ("Druck"=w292:dbl)  [unwired: 5 in, 5 out]
      n141 = Number To Fractional String(number=w292, precision (6)=i16 3 ("Genauigkeit (6)")) -> (F-format string=w287:string)  [unwired: 2 in]
      n142 = Number To Fractional String(number=w290, precision (6)=i16 0 ("Genauigkeit (6)")) -> (F-format string=w285:string)  [unwired: 2 in]
      n143 = Number To Fractional String(number=w288, precision (6)=i16 1 ("Genauigkeit (6)")) -> (F-format string=w286:string)  [unwired: 2 in]
      n144 = Build Array(w287, w285, w286) -> (w296:string[])
      n145 = for {
        tunnel: w296 -> [w302] mode=indexing
        shift-right: [w303] -> w295
        shift-left: w294 -> [w305]
        n146 = call <vilib>:"Space Constant.vi"() -> ("String"=w304:string)
        n147 = Concatenate Strings(w305, w304, w302) -> (w303:string)
      }
    }
    frame "ADUF" {
      n148 = call "Zustandsfehlerinformation.vi"("Aktionen"=Aktionen_Zustandsfehlerinformation."OK", "String"=w314) -> ("String"=w310:string)  [unwired: 9 in]
      n149 = call "FGV cRIO-Daten.vi"("Aktion"=enum16{"lesen", "schreiben"}."lesen") -> ("Analog Input"=w313:T27)  [unwired: 9 in, 9 out]
      n150 = Unbundle By Name(w313) -> ("AI0: Durchfluss FT-IR"=w309:sgl)
      n151 = Number To Fractional String(number=w309, precision (6)=i16 1 ("Genauigkeit (6)")) -> (F-format string=w306:string)  [unwired: 2 in]
      n152 = call <vilib>:"Space Constant.vi"() -> ("String"=w307:string)
      n153 = Concatenate Strings(w310, w307, w306) -> (w311:string)
    }
    frame "AGID" {
      n154 = call "Zustandsfehlerinformation.vi"("Aktionen"=Aktionen_Zustandsfehlerinformation."OK", "String"=w321) -> ("String"=w318:string)  [unwired: 9 in]
      n155 = call "FGV System Konstanten.vi"("Aktionen"=Aktioen_FGV_System_Konstanten."lesen") -> ("LanguageList"=w317:string)  [unwired: 6 in, 4 out]
      n156 = call <vilib>:"Space Constant.vi"() -> ("String"=w320:string)
      n157 = Concatenate Strings(w318, w320, w317) -> (w316:string)
    }
    frame "AVER" {
      n158 = call "Zustandsfehlerinformation.vi"("Aktionen"=Aktionen_Zustandsfehlerinformation."OK", "String"=w329) -> ("String"=w326:string)  [unwired: 9 in]
      n159 = call "FGV System Konstanten.vi"("Aktionen"=Aktioen_FGV_System_Konstanten."lesen") -> ("Cluster out"=w324:T21)  [unwired: 6 in, 4 out]
      n160 = Unbundle By Name(w324) -> ("Software Version"=w323:string)
      n161 = call <vilib>:"Space Constant.vi"() -> ("String"=w328:string)
      n162 = Concatenate Strings(w326, w328, w323) -> (w325:string)
    }
    frame "ALEC" {
      n163 = call "Zustandsfehlerinformation.vi"("Aktionen"=Aktionen_Zustandsfehlerinformation."OK", "String"=w344) -> ("String"=w343:string)  [unwired: 9 in]
      n164 = call "Status Dichtheitstest.vi"("Aktionen"=Status_Dichtheitstest_Aktionen."lesen") -> ("Fehler"=w332:bool, "läuft?"=w336:bool, "Anstieg"=w341:sgl)  [unwired: 6 in, 2 out]
      n165 = Or(x=w336, y=w332) -> (x .or. y?=w335:bool)
      n166 = Number To Decimal String(number=w341) -> (decimal integer string=w340:string)  [unwired: 1 in]
      n167 = call <vilib>:"Space Constant.vi"() -> ("String"=w339:string)
      n168 = Concatenate Strings(w343, w339, w340) -> (w338:string)
      n169 = Select(t="error", s=w332, f="busy") -> (s? t:f=w331:string)
      n170 = case shown="True" w335 {
        tunnel: w338 -> [w346 w349]
        tunnel: [w346 w347] -> w337
        tunnel: w331 -> [_ w348]
        frame False {
        }
        frame True {
          n171 = call <vilib>:"Space Constant.vi"() -> ("String"=w350:string)
          n172 = Concatenate Strings(w349, w350, w348) -> (w347:string)
        }
      }
    }
    frame "ALES" {
      n173 = call "FGV Erweiterte Konfig.vi"("Aktion"=FGV_PID_Aktionen."Lesen") -> ("Sonstige"=w357:T28)  [unwired: 5 in, 5 out]
      n174 = call "Zustandsfehlerinformation.vi"("Aktionen"=Aktionen_Zustandsfehlerinformation."OK", "String"=w365) -> ("String"=w362:string)  [unwired: 9 in]
      n175 = Unbundle By Name(w357) -> ("Dichtheitstest Zeit"=w354:sgl, "Dichtheitstest Abfall"=w353:sgl, "Dichtheitstest Umfang"=w352:T31)
      n176 = Number To Fractional String(number=w354, precision (6)=i16 0 ("Genauigkeit (6)")) -> (F-format string=w351:string)  [unwired: 2 in]
      n177 = Number To Fractional String(number=w353, precision (6)=i16 0 ("Genauigkeit (6)")) -> (F-format string=w358:string)  [unwired: 2 in]
      n178 = Number To Fractional String(number=w352, precision (6)=i16 0 ("Genauigkeit (6)")) -> (F-format string=w359:string)  [unwired: 2 in]
      n179 = Build Array(w351, w358, w359) -> (w364:string[])
      n180 = for {
        tunnel: w364 -> [w367] mode=indexing
        shift-right: [w368] -> w363
        shift-left: w362 -> [w370]
        n181 = call <vilib>:"Space Constant.vi"() -> ("String"=w369:string)
        n182 = Concatenate Strings(w370, w369, w367) -> (w368:string)
      }
    }
    frame "ANOS" {
      n183 = call "Zustandsfehlerinformation.vi"("Aktionen"=Aktionen_Zustandsfehlerinformation."OK", "String"=w376) -> ("String"=w375:string)  [unwired: 9 in]
      n184 = call "FGV FT-IR Parameter.vi"("Aktion"=FGV_FT-IR_Aktionen."lesen") -> ("NoOfScan"=w371:u32)  [unwired: 11 in, 7 out]
      n185 = call <vilib>:"Space Constant.vi"() -> ("String"=w374:string)
      n186 = Number To Decimal String(number=w371) -> (decimal integer string=w373:string)  [unwired: 1 in]
      n187 = Concatenate Strings(w375, w374, w373) -> (w378:string)
    }
    frame "ALNB" {
      n188 = call "Zustandsfehlerinformation.vi"("Aktionen"=Aktionen_Zustandsfehlerinformation."OK", "String"=w385) -> ("String"=w384:string)  [unwired: 9 in]
      n189 = call "FGV Erweiterte Konfig.vi"("Aktion"=FGV_PID_Aktionen."Lesen") -> ("Sonstige"=w381:T28)  [unwired: 5 in, 5 out]
      n190 = Unbundle By Name(w381) -> ("Befüllung aktiv"=w379:T30)
      n191 = call <vilib>:"Space Constant.vi"() -> ("String"=w383:string)
      n192 = Number To Decimal String(number=w379) -> (decimal integer string=w382:string)  [unwired: 1 in]
      n193 = Concatenate Strings(w384, w383, w382) -> (w387:string)
    }
    frame "ADFT" {
      n194 = call "FGV Anlagengrenzwerte.vi"("Aktion"=FGV_Anlagengrenzwerte_Aktionen."Lesen") -> ("Anlagen-Grenzwerte Anzeige"=w391:T32)  [unwired: 1 in, 9 out]
      n195 = call "Zustandsfehlerinformation.vi"("Aktionen"=Aktionen_Zustandsfehlerinformation."OK", "String"=w395) -> ("String"=w394:string)  [unwired: 9 in]
      n196 = Unbundle By Name(w391) -> ("Durchfluss FT-IR:.Sollwert"=w390:sgl)
      n197 = call <vilib>:"Space Constant.vi"() -> ("String"=w393:string)
      n198 = Number To Fractional String(number=w390, precision (6)=i16 1 ("Genauigkeit (6)")) -> (F-format string=w388:string)  [unwired: 2 in]
      n199 = Concatenate Strings(w394, w393, w388) -> (w397:string)
    }
    frame "ABST" {
      n200 = call "Zustandsfehlerinformation.vi"("Aktionen"=Aktionen_Zustandsfehlerinformation."OK", "String"=w409) -> ("String"=w406:string)  [unwired: 9 in]
      n201 = call "FGV cRIO-Daten.vi"("Aktion"=enum16{"lesen", "schreiben"}."lesen") -> ("PID Stellwerte"=w398:i16[])  [unwired: 9 in, 9 out]
      n202 = Index Array(array=w398) -> (element #1=w399:i16, element #2=w400:i16)  [unwired: 2 in]
      n203 = Number To Fractional String(number=w399, precision (6)=i16 1 ("Genauigkeit (6)")) -> (F-format string=w403:string)  [unwired: 2 in]
      n204 = Number To Fractional String(number=w400, precision (6)=i16 1 ("Genauigkeit (6)")) -> (F-format string=w402:string)  [unwired: 2 in]
      n205 = Build Array(w403, w402) -> (w408:string[])
      n206 = for {
        tunnel: w408 -> [w411] mode=indexing
        shift-right: [w412] -> w407
        shift-left: w406 -> [w414]
        n207 = call <vilib>:"Space Constant.vi"() -> ("String"=w413:string)
        n208 = Concatenate Strings(w414, w413, w411) -> (w412:string)
      }
    }
    frame "SECO" {
      n209 = call "Setze Zustand.vi"("AK Befehl"=w417, "Zustand"=Zustaende."Eco") -> ("Antwort String"=w416:string)  [unwired: 8 in, 1 out]
    }
    frame "SPAU" {
      n210 = call "Setze Zustand.vi"("AK Befehl"=w420, "Zustand"=Zustaende."Pause") -> ("Antwort String"=w419:string)  [unwired: 8 in, 1 out]
    }
    frame "STBY" {
      n211 = call "Setze Zustand.vi"("AK Befehl"=w423, "Zustand"=Zustaende."Standby") -> ("Antwort String"=w422:string)  [unwired: 8 in, 1 out]
    }
    frame "SMGA" {
      n212 = call "Setze Zustand.vi"("AK Befehl"=w426, "Zustand"=Zustaende."Messen") -> ("Antwort String"=w425:string)  [unwired: 8 in, 1 out]
    }
    frame "SSPL" {
      n213 = Index Array(array=w428, index=2 ("Index")) -> (element=w432:string)
      n214 = Decimal String To Number(string=w432) -> (number=w431:i32)  [unwired: 2 in, 1 out]
      n215 = Divide(x=w431, y=10) -> (x/y=w429:dbl)
      n216 = To Single Precision Float(number=w429) -> (single precision float=w427:sgl)
      n217 = call "Setze Zustand.vi"("Zeit"=w427, "AK Befehl"=w436, "Zustand"=Zustaende."Spülen Leitung") -> ("Antwort String"=w435:string)  [unwired: 7 in, 1 out]
    }
    frame "SRUC" {
      n218 = Index Array(array=w438, index=2 ("Index")) -> (element=w442:string)
      n219 = Decimal String To Number(string=w442) -> (number=w441:i32)  [unwired: 2 in, 1 out]
      n220 = Divide(x=w441, y=10) -> (x/y=w439:dbl)
      n221 = To Single Precision Float(number=w439) -> (single precision float=w437:sgl)
      n222 = call "Setze Zustand.vi"("Zeit"=w437, "AK Befehl"=w446, "Zustand"=Zustaende."Spülen Filter") -> ("Antwort String"=w445:string)  [unwired: 7 in, 1 out]
    }
    frame "SSPR" {
      n223 = call "Setze Zustand.vi"("Befehl nicht vorhanden!"=TRUE, "AK Befehl"=w450, "Zustand"=Zustaende."Standby") -> ("Antwort String"=w449:string)  [unwired: 7 in, 1 out]
    }
    frame "SNGA" {
      n224 = Index Array(array=w458, index=2 ("Index")) -> (element=w456:string)
      n225 = Decimal String To Number(string=w456) -> (number=w455:i32)  [unwired: 2 in, 1 out]
      n226 = Divide(x=w455, y=10) -> (x/y=w453:dbl)
      n227 = To Single Precision Float(number=w453) -> (single precision float=w451:sgl)
      n228 = call "Setze Zustand.vi"("Zeit"=w451, "AK Befehl"=w460, "Zustand"=Zustaende."0-Gas") -> ("Antwort String"=w459:string)  [unwired: 7 in, 1 out]
    }
    frame "SNGF" {
      n229 = call "Setze Zustand.vi"("Befehl nicht vorhanden!"=TRUE, "AK Befehl"=w464, "Zustand"=Zustaende."Standby") -> ("Antwort String"=w463:string)  [unwired: 7 in, 1 out]
    }
    frame "SMAN" {
      n230 = call "FGV-Funktionstasten.vi"("Aktion"=Funktionstasten-Aktion."Lesen") -> ("Betriebsart"=w470:T19)  [unwired: 7 in, 7 out]
      n231 = Equal?(x=w470, y=Betriebsart."Remote" ("Betriebsart")) -> (x = y?=w467:bool)
      n232 = case shown="True" w467 {
        tunnel: w466 -> [w473 w476]
        tunnel: [w471 w475] -> w465
        frame False {
          n233 = call "Zustandsfehlerinformation.vi"("Aktionen"=Aktionen_Zustandsfehlerinformation."Offline", "String"=w473) -> ("String"=w471:string)  [unwired: 9 in]
        }
        frame True {
          n234 = call "Zustandsfehlerinformation.vi"("Aktionen"=Aktionen_Zustandsfehlerinformation."OK", "String"=w476) -> ("String"=w475:string)  [unwired: 9 in]
          n235 = call "FGV-Funktionstasten.vi"("Aktion"=Funktionstasten-Aktion."Manuell") -> ()  [unwired: 7 in, 8 out]
        }
      }
    }
    frame "SREM" {
      n236 = call "Zustandsfehlerinformation.vi"("Aktionen"=Aktionen_Zustandsfehlerinformation."OK", "String"=w479) -> ("String"=w478:string)  [unwired: 9 in]
      n237 = call "FGV-Funktionstasten.vi"("Aktion"=Funktionstasten-Aktion."Remote") -> ()  [unwired: 7 in, 8 out]
    }
    frame "SEMB" {
      n238 = call "FGV-Funktionstasten.vi"("Aktion"=Funktionstasten-Aktion."Lesen") -> ("Betriebsart"=w487:T19)  [unwired: 7 in, 7 out]
      n239 = Equal?(x=w487, y=Betriebsart."Remote" ("Betriebsart")) -> (x = y?=w488:bool)
      n240 = case shown="True" w488 {
        tunnel: w484 -> [w490 w502]
        tunnel: [w489 w501] -> w483
        tunnel: w482 -> [_ w500]
        frame False {
          n241 = call "Zustandsfehlerinformation.vi"("Aktionen"=Aktionen_Zustandsfehlerinformation."Offline", "String"=w490) -> ("String"=w489:string)  [unwired: 9 in]
        }
        frame True {
          n242 = Index Array(array=w500, index=2 ("Index")) -> (element=w498:string)
          n243 = call "Zustandsfehlerinformation.vi"("Aktionen"=Aktionen_Zustandsfehlerinformation."OK", "String"=w502) -> ("String"=w501:string)  [unwired: 9 in]
          n244 = Decimal String To Number(string=w498, offset=1 ("Offset (0)")) -> (number=w494:i32)  [unwired: 1 in, 1 out]
          n245 = call "Gespeicherte Werte.vi"("Aktionen"=Aktionen_Gespeicherte_Werte."lesen") -> ("Diverse Werte"=w493:T23)  [unwired: 6 in, 4 out]
          n246 = Bundle By Name(cluster=w493, "Kalibriergaseingang"=w494) -> (w492:T23)
          n247 = call "Gespeicherte Werte.vi"("Aktionen"=Aktionen_Gespeicherte_Werte."Diverse", "Diverse Werte"=w492) -> ()  [unwired: 5 in, 5 out]
        }
      }
    }
    frame "SEKA" {
      n248 = call "FGV-Funktionstasten.vi"("Aktion"=Funktionstasten-Aktion."Lesen") -> ("Betriebsart"=w509:T19)  [unwired: 7 in, 7 out]
      n249 = Equal?(x=w509, y=Betriebsart."Remote" ("Betriebsart")) -> ()  [unwired: 1 out]
      n250 = call "Zustandsfehlerinformation.vi"("Aktionen"=Aktionen_Zustandsfehlerinformation."OK", "String"=w506) -> ("String"=w505:string)  [unwired: 9 in]
    }
    frame "SATK" {
      n251 = call "Setze Zustand.vi"("AK Befehl"=w511, "Zustand"=Zustaende."Kalibrieren") -> ("Antwort String"=w510:string)  [unwired: 8 in, 1 out]
    }
    frame "SENT" {
      n252 = call "FGV-Funktionstasten.vi"("Aktion"=Funktionstasten-Aktion."Lesen") -> ("Betriebsart"=w518:T19)  [unwired: 7 in, 7 out]
      n253 = Equal?(x=w518, y=Betriebsart."Remote" ("Betriebsart")) -> (x = y?=w519:bool)
      n254 = case shown="True" w519 {
        tunnel: w515 -> [w521 w533]
        tunnel: [w520 w532] -> w514
        tunnel: w513 -> [_ w531]
        frame False {
          n255 = call "Zustandsfehlerinformation.vi"("Aktionen"=Aktionen_Zustandsfehlerinformation."Offline", "String"=w521) -> ("String"=w520:string)  [unwired: 9 in]
        }
        frame True {
          n256 = Index Array(array=w531, index=2 ("Index")) -> (element=w529:string)
          n257 = call "Zustandsfehlerinformation.vi"("Aktionen"=Aktionen_Zustandsfehlerinformation."OK", "String"=w533) -> ("String"=w532:string)  [unwired: 9 in]
          n258 = Decimal String To Number(string=w529) -> (number=w523:i32)  [unwired: 2 in, 1 out]
          n259 = call "FGV-Funktionstasten.vi"("Samplepoint"=w523, "Aktion"=Funktionstasten-Aktion."Samplepoint") -> ()  [unwired: 6 in, 8 out]
          n260 = call "Gespeicherte Werte.vi"("Aktionen"=Aktionen_Gespeicherte_Werte."lesen") -> ("Diverse Werte"=w526:T23)  [unwired: 6 in, 4 out]
          n261 = Bundle By Name(cluster=w526, "SamplePoint"=w523) -> (w525:T23)
          n262 = call "Gespeicherte Werte.vi"("Aktionen"=Aktionen_Gespeicherte_Werte."Diverse", "Diverse Werte"=w525) -> ()  [unwired: 5 in, 5 out]
        }
      }
    }
    frame "STRG" {
      n263 = call "FGV-Funktionstasten.vi"("Aktion"=Funktionstasten-Aktion."Lesen") -> ("Betriebsart"=w540:T19)  [unwired: 7 in, 7 out]
      n264 = Equal?(x=w540, y=Betriebsart."Remote" ("Betriebsart")) -> (x = y?=w541:bool)
      n265 = case shown="True" w541 {
        tunnel: w537 -> [w543 w550]
        tunnel: [w542 w549] -> w536
        tunnel: w535 -> [_ w548]
        frame False {
          n266 = call "Zustandsfehlerinformation.vi"("Aktionen"=Aktionen_Zustandsfehlerinformation."Offline", "String"=w543) -> ("String"=w542:string)  [unwired: 9 in]
        }
        frame True {
          n267 = Index Array(array=w548, index=2 ("Index")) -> (element=w546:string)
          n268 = Empty String/Path?(string/path=w546) -> (empty?=w545:bool)
          n269 = case shown="False" w545 {
            tunnel: w550 -> [w557 w570]
            tunnel: [w556 w569] -> w549
            tunnel: w546 -> [w555 _]
            frame False {
              n270 = Decimal String To Number(string=w555) -> (number=w552:i32)  [unwired: 2 in, 1 out]
              n271 = In Range and Coerce(upper limit=2 ("Obergrenze"), x=w552, lower limit=0 ("Untergrenze")) -> (In Range?=w551:bool)  [unwired: 1 out]
              n272 = case shown="True" w551 {
                tunnel: w557 -> [w559 w567]
                tunnel: [w558 w566] -> w556
                tunnel: w552 -> [_ w561]
                frame False {
                  n273 = call "Zustandsfehlerinformation.vi"("Aktionen"=Aktionen_Zustandsfehlerinformation."Datenfehler", "String"=w559) -> ("String"=w558:string)  [unwired: 9 in]
                }
                frame True {
                  # "Wenn informationen da sind, dann übergeben!"
                  n274 = call "FGV Trigger.vi"("Aktion"=Aktionen_Trigger."lesen") -> ("Triggerereignis neu"=w563:T34)  [unwired: 7 in, 3 out]
                  n275 = Bundle By Name(cluster=w563, "Trigger verwenden"=w561) -> (w562:T34)
                  n276 = call "Zustandsfehlerinformation.vi"("Aktionen"=Aktionen_Zustandsfehlerinformation."OK", "String"=w567) -> ("String"=w566:string)  [unwired: 9 in]
                  n277 = call "FGV Trigger.vi"("Aktion"=Aktionen_Trigger."ALLE schreiben", "Triggerereignis"=w562) -> ()  [unwired: 6 in, 4 out]
                }
              }
            }
            frame True {
              # "Wenn nur STRG dann Trigger setzen!!!"
              n278 = call "FGV Trigger.vi"("Aktion"=Aktionen_Trigger."Trigger prüfen", "Trigger setzen"=TRUE) -> ()  [unwired: 6 in, 4 out]
              n279 = call "Zustandsfehlerinformation.vi"("Aktionen"=Aktionen_Zustandsfehlerinformation."OK", "String"=w570) -> ("String"=w569:string)  [unwired: 9 in]
            }
          }
        }
      }
    }
    frame "SLEC" {
      n280 = call "FGV-Funktionstasten.vi"("Aktion"=Funktionstasten-Aktion."Lesen") -> ("ausgewählte Funktion"=w574:T10, "Betriebsart"=w579:T19)  [unwired: 7 in, 6 out]
      n281 = Equal?(x=w579, y=Betriebsart."Remote" ("Betriebsart")) -> (x = y?=w580:bool)
      n282 = case shown="True" w580 {
        tunnel: w576 -> [w582 w588]
        tunnel: [w581 w587] -> w575
        tunnel: w574 -> [_ w586]
        frame False {
          n283 = call "Zustandsfehlerinformation.vi"("Aktionen"=Aktionen_Zustandsfehlerinformation."Offline", "String"=w582) -> ("String"=w581:string)  [unwired: 9 in]
        }
        frame True {
          n284 = Equal?(x=w586, y=Zustaende."Standby") -> (x = y?=w584:bool)
          n285 = case shown="True" w584 {
            tunnel: w588 -> [w591 w593]
            tunnel: [w590 w592] -> w587
            frame False {
              n286 = call "Zustandsfehlerinformation.vi"("Aktionen"=Aktionen_Zustandsfehlerinformation."Datenfehler", "String"=w591) -> ("String"=w590:string)  [unwired: 9 in]
            }
            frame True {
              n287 = flat-sequence {
                frame #0 {
                  n288 = call "FGV Erweiterte Konfig.vi"("Aktion"=FGV_PID_Aktionen."Dichtheitstest", "Dichtheitstest?"=TRUE) -> ()  [unwired: 5 in, 5 out]
                }
                frame #1 {
                  n289 = vi-ref "Erweiterte Konfig.lvlib:Dichtheitstest.vi"() -> (w597:refnum<vi>)
                  n290 = call "VI Pop Up.vi"("VI Referenz"=w597) -> ()  [unwired: 10 in, 1 out]
                }
              }
              n291 = call "Zustandsfehlerinformation.vi"("Aktionen"=Aktionen_Zustandsfehlerinformation."OK", "String"=w593) -> ("String"=w592:string)  [unwired: 9 in]
            }
          }
        }
      }
    }
    frame "SLES" {
      n292 = call "FGV-Funktionstasten.vi"("Aktion"=Funktionstasten-Aktion."Lesen") -> ("Betriebsart"=w603:T19)  [unwired: 7 in, 7 out]
      n293 = Equal?(x=w603, y=Betriebsart."Remote" ("Betriebsart")) -> (x = y?=w604:bool)
      n294 = case shown="True" w604 {
        tunnel: w600 -> [w606 w639]
        tunnel: [w605 w638] -> w599
        tunnel: w598 -> [_ w637]
        frame False {
          n295 = call "Zustandsfehlerinformation.vi"("Aktionen"=Aktionen_Zustandsfehlerinformation."Offline", "String"=w606) -> ("String"=w605:string)  [unwired: 9 in]
        }
        frame True {
          n296 = Index Array(array=w637, index #1=2 ("Index"), index #2=3 ("Index"), index #3=4 ("Index")) -> (element #1=w611:string, element #2=w612:string, element #3=w613:string)
          n297 = Empty String/Path?(string/path=w611) -> (empty?=w616:bool)
          n298 = Empty String/Path?(string/path=w612) -> (empty?=w615:bool)
          n299 = Empty String/Path?(string/path=w613) -> (empty?=w614:bool)
          n300 = Decimal String To Number(string=w611) -> (number=w633:i32)  [unwired: 2 in, 1 out]
          n301 = Decimal String To Number(string=w612) -> (number=w629:i32)  [unwired: 2 in, 1 out]
          n302 = Decimal String To Number(string=w613) -> (number=w624:i32)  [unwired: 2 in, 1 out]
          n303 = Not(x=w616) -> (.not. x?=w610:bool)
          n304 = Not(x=w615) -> (.not. x?=w609:bool)
          n305 = Not(x=w614) -> (.not. x?=w608:bool)
          n306 = In Range and Coerce(upper limit=101 ("Obergrenze"), x=w633, lower limit=1 ("Untergrenze")) -> (coerced(x)=w619:i32, In Range?=w621:bool)
          n307 = In Range and Coerce(upper limit=101 ("Obergrenze"), x=w629, lower limit=1 ("Untergrenze")) -> (coerced(x)=w618:i32, In Range?=w622:bool)
          n308 = In Range and Coerce(upper limit=3 ("Obergrenze"), x=w624, lower limit=0 ("Untergrenze")) -> (coerced(x)=w617:i32, In Range?=w623:bool)
          n309 = Compound Arithmetic op=AND(w621, w622, w623, w610, w609, w608) -> (w620:bool)
          n310 = case shown="True" w620 {
            tunnel: [Aktionen_Zustandsfehlerinformation."Datenfehler" ("Aktionen") Aktionen_Zustandsfehlerinformation."OK" ("Aktionen")] -> w632
            tunnel: w619 -> [_ w643]
            tunnel: w618 -> [_ w642]
            tunnel: w617 -> [_ w641]
            frame False {
            }
            frame True {
              n311 = call "FGV Erweiterte Konfig.vi"("Aktion"=FGV_PID_Aktionen."Lesen") -> ("Sonstige"=w646:T28)  [unwired: 5 in, 5 out]
              n312 = Bundle By Name(cluster=w646, "Dichtheitstest Zeit"=w643, "Dichtheitstest Abfall"=w642, "Dichtheitstest Umfang"=w641) -> (w647:T28)
              n313 = call "FGV Erweiterte Konfig.vi"("Aktion"=FGV_PID_Aktionen."Schreiben Sonstige", "Sonstige"=w647) -> ()  [unwired: 4 in, 6 out]
            }
          }
          n314 = call "Zustandsfehlerinformation.vi"("Aktionen"=w632, "String"=w639) -> ("String"=w638:string)  [unwired: 9 in]
        }
      }
    }
    frame "SLNB" {
      n315 = call "FGV-Funktionstasten.vi"("Aktion"=Funktionstasten-Aktion."Lesen") -> ("Betriebsart"=w654:T19)  [unwired: 7 in, 7 out]
      n316 = Equal?(x=w654, y=Betriebsart."Remote" ("Betriebsart")) -> (x = y?=w655:bool)
      n317 = case shown="True" w655 {
        tunnel: w651 -> [w657 w672]
        tunnel: [w656 w671] -> w650
        tunnel: w649 -> [_ w670]
        frame False {
          n318 = call "Zustandsfehlerinformation.vi"("Aktionen"=Aktionen_Zustandsfehlerinformation."Offline", "String"=w657) -> ("String"=w656:string)  [unwired: 9 in]
        }
        frame True {
          # "0 oder 1"
          n319 = Index Array(array=w670, index=2 ("Index")) -> (element=w661:string)
          n320 = Decimal String To Number(string=w661) -> (number=w666:i32)  [unwired: 2 in, 1 out]
          n321 = Empty String/Path?(string/path=w661) -> (empty?=w660:bool)
          n322 = In Range and Coerce(upper limit=2 ("Obergrenze"), x=w666, lower limit=0 ("Untergrenze")) -> (coerced(x)=w662:i32, In Range?=w664:bool)
          n323 = Not(x=w660) -> (.not. x?=w659:bool)
          n324 = And(x=w664, y=w659) -> (x .and. y?=w663:bool)
          n325 = case shown="True" w663 {
            tunnel: [Aktionen_Zustandsfehlerinformation."Datenfehler" ("Aktionen") Aktionen_Zustandsfehlerinformation."OK" ("Aktionen")] -> w665
            tunnel: w662 -> [_ w674]
            frame False {
            }
            frame True {
              n326 = call "FGV Erweiterte Konfig.vi"("Aktion"=FGV_PID_Aktionen."Lesen") -> ("Sonstige"=w677:T28)  [unwired: 5 in, 5 out]
              n327 = Bundle By Name(cluster=w677, "Befüllung aktiv"=w674) -> (w678:T28)
              n328 = call "FGV Erweiterte Konfig.vi"("Aktion"=FGV_PID_Aktionen."Schreiben Sonstige", "Sonstige"=w678) -> ()  [unwired: 4 in, 6 out]
            }
          }
          n329 = call "Zustandsfehlerinformation.vi"("Aktionen"=w665, "String"=w672) -> ("String"=w671:string)  [unwired: 9 in]
        }
      }
    }
    frame "SNOS" {
      n330 = call "FGV-Funktionstasten.vi"("Aktion"=Funktionstasten-Aktion."Lesen") -> ("Betriebsart"=w685:T19)  [unwired: 7 in, 7 out]
      n331 = Equal?(x=w685, y=Betriebsart."Remote" ("Betriebsart")) -> (x = y?=w686:bool)
      n332 = case shown="True" w686 {
        tunnel: w682 -> [w688 w700]
        tunnel: [w687 w699] -> w681
        tunnel: w680 -> [_ w698]
        frame False {
          n333 = call "Zustandsfehlerinformation.vi"("Aktionen"=Aktionen_Zustandsfehlerinformation."Offline", "String"=w688) -> ("String"=w687:string)  [unwired: 9 in]
        }
        frame True {
          n334 = Index Array(array=w698, index=2 ("Index")) -> (element=w696:string)
          n335 = Decimal String To Number(string=w696) -> (number=w693:i32)  [unwired: 2 in, 1 out]
          n336 = In Range and Coerce(upper limit=101 ("Obergrenze"), x=w693, lower limit=1 ("Untergrenze")) -> (coerced(x)=w692:i32, In Range?=w691:bool)
          n337 = case shown="True" w691 {
            tunnel: w692 -> [_ w702]
            tunnel: [Aktionen_Zustandsfehlerinformation."Datenfehler" ("Aktionen") Aktionen_Zustandsfehlerinformation."OK" ("Aktionen")] -> w690
            frame False {
            }
            frame True {
              n338 = flat-sequence {
                tunnel: w702 -> [w704]
                frame #0 {
                  n339 = call "FGV FT-IR Parameter.vi"("NoOfScan neu"=w704, "Aktion"=FGV_FT-IR_Aktionen."NOS setzen") -> ("NoOfScan"=w705:u32)  [unwired: 10 in, 7 out]
                  n340 = call "TOOLweb SET ftirScans.vi"("ftirScans"=w705) -> ()  [unwired: 2 in, 5 out]
                }
                frame #1 {
                  n341 = call "Queue LogFile.vi"() -> ("error out"=w710:errorcluster, "Queue (Ausgang)"=w709:refnum<queue>)  [unwired: 6 in]
                  n342 = call "FGV Messdaten.vi"("Aktionen"=Aktionen_FGV_Messdaten."löschen") -> ()  [unwired: 6 in, 9 out]
                  n343 = Flush Queue(queue=w709, error in (no error)=w710) -> (error out=w707:errorcluster)  [unwired: 2 out]
                  n344 = call <vilib>:"Clear Errors.vi"("error in (no error)"=w707) -> ()  [unwired: 5 in, 2 out]
                }
              }
            }
          }
          n345 = call "Zustandsfehlerinformation.vi"("Aktionen"=w690, "String"=w700) -> ("String"=w699:string)  [unwired: 9 in]
        }
      }
    }
  }
  "String für schreiben" <- w5
